vi "Initialise QMH CORE.vi"(8 "Error in":errorcluster, 11 "External Event":refnum<user-event>) -> (0 "Error out":errorcluster, 2 "Event Registration Refnum":refnum<event-registration>, 3 "Queue Data":T1)   [LabVIEW 2018, in "QMH CORE.lvlib"]
uses:
  QMH/QMH CORE.lvlib
  Type Defs/EventsAndQueues--cluster.ctl
  Queue Messaging/Type Defs/Queue Message--cluster.ctl
  Event Messaging/Type Defs/Event Message--cluster.ctl
  Queue Messaging/Queue Messaging.lvlib
  Event Messaging/Event Messaging.lvlib
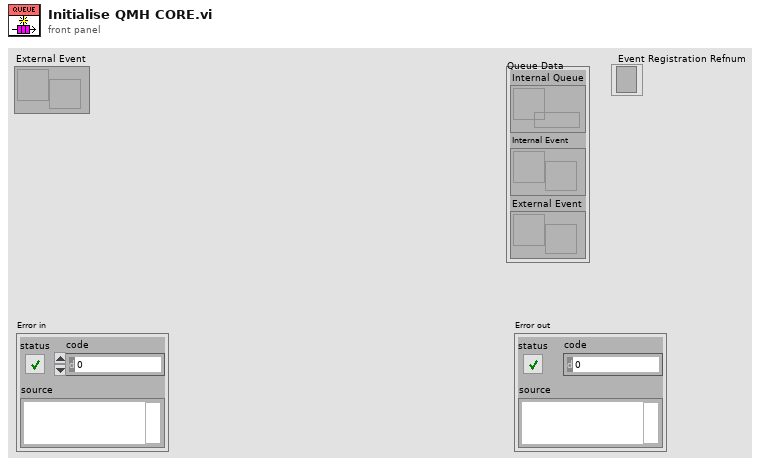
[diagram p1: front panel]
types:
  T1 = typedef "QMH CORE.lvlib/EventsAndQueues--cluster.ctl" = cluster{"Internal Queue":refnum<queue>, "Internal Event":refnum<user-event>, "External Event":refnum<user-event>}
  T2 = typedef "Queue Messaging.lvlib/Queue Message--cluster.ctl" = cluster{"Cmd":string, "Data":variant}
  T3 = typedef "Event Messaging.lvlib/Event Message--cluster.ctl" = cluster{"Cmd":string, "Data":variant}
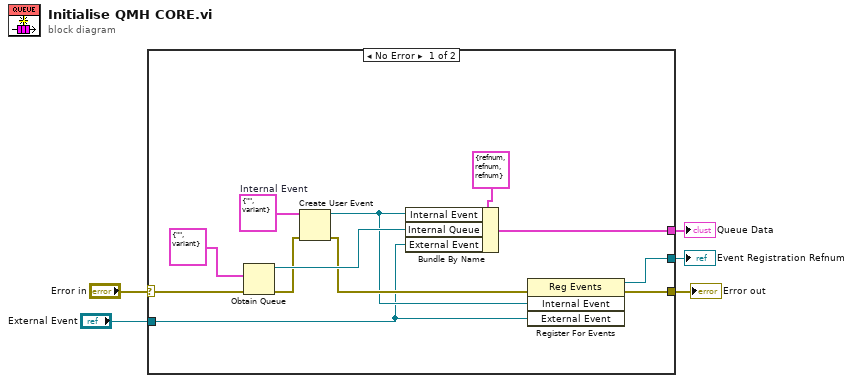
[diagram p0: block diagram]
diagram:
  n1 = case shown="No Error" "Error in" {
    selector: "Error in" -> [w16 w18]
    tunnel: [w8 w18] -> w4
    tunnel: [w13 _] -> w3
    tunnel: "External Event" -> [w6 _]
    tunnel: [w10 _] -> w1
    frame No Error {
      w11 = T3 {"Cmd"="", "Data"=variant}  # Internal Event
      n2 = Obtain Queue(element data type=T2 {"Cmd"="", "Data"=variant} ("Message"), error in (no error)=w16) -> (queue out=w14:refnum<queue>, error out=w12:errorcluster)  [unwired: 3 in, 1 out]
      n3 = Create User Event(user event datatype=w11, error in=w12) -> (user event=w7:refnum<user-event>, error out=w9:errorcluster)
      n4 = Bundle By Name(cluster=T1 {"Internal Queue"=refnum, "Internal Event"=refnum, "External Event"=refnum}, "Internal Event"=w7, "Internal Queue"=w14, "External Event"=w6) -> (w13:T1)
      n5 = register-events(error in=w9, w7, w6) -> (reference out=w10:refnum<event-registration>, error out=w8:errorcluster)  [unwired: 1 in]
    }
    frame Error {
    }
  }
  "Error out" <- w4
  "Queue Data" <- w3
  "Event Registration Refnum" <- w1
